vi "Queue Actor.vi"(8 "Queue Caller":map{string, refnum<data-value>}(c390), 9 "Queue of Queue Self":refnum<queue>, 10 "Queue Self Alias":string, 11 "Queue Actor":refnum<class "Queue Actor.lvclass">) -> ()   [LabVIEW 2021, in "jettl Queue Actor.lvlib" / "jettl Queue Actor.lvclass"]
uses:
  jettl Queue Actor.lvclass
  jettl Queue Actor.lvlib
  Actor/Msgs/Queue Last Ack/Queue Last Ack Msg/Queue Last Ack Msg.lvclass
  Actor/Msgs/Setup/Setup Msg/Setup Msg.lvclass
  Actor/Queue Actor/Queue Actor.lvclass
  Actor/Msg/Msg.lvclass
  C:/git/jettl/src/Actor/Actor/Actor.lvclass
  C:/git/jettl/src/Actor/Msgs/Setup/Setup/Setup.lvclass
  C:/git/jettl/src/Actor/Msgs/Teardown/Teardown/Teardown.lvclass
  C:/git/jettl/src/Actor/Queue Actor/Queue Actor.lvclass
  C:/git/jettl/src/Actor/Msgs/Event Create/Event Create/Event Create.lvclass
  C:/git/jettl/src/Actor/Msgs/Event Last Ack/Event Last Ack/Event Last Ack.lvclass
  C:/git/jettl/src/Actor/Msgs/Queue Create/Queue Create/Queue Create.lvclass
  C:/git/jettl/src/Actor/Msgs/Queue Last Ack/Queue Last Ack/Queue Last Ack.lvclass
  C:/git/jettl/src/jettl/jettl Queue Actor/jettl Queue Actor/jettl Queue Actor.lvclass
  C:/git/jettl/src/Actor/Msgs/Setup/Setup Msg/Setup Msg.lvclass
  C:/git/jettl/src/Actor/Msg/Msg.lvclass
  C:/git/jettl/src/Actor/Msgs/Queue Last Ack/Queue Last Ack Msg/Queue Last Ack Msg.lvclass
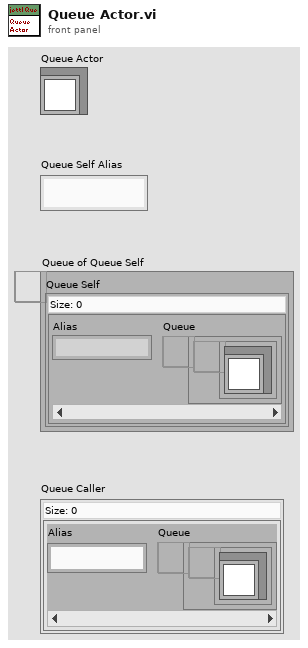
[diagram p1: front panel]
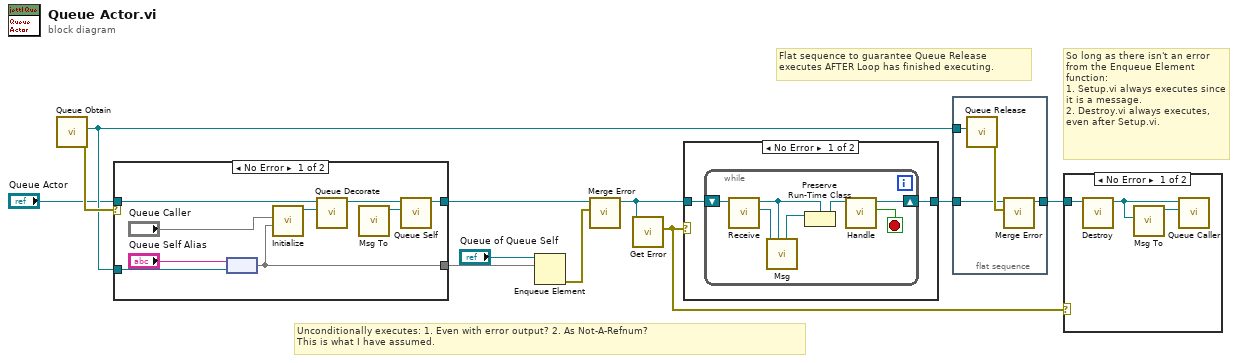
[diagram p0: block diagram]
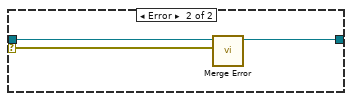
[diagram p3: hidden frame]
diagram:
  # "Flat sequence to guarantee Queue Release executes AFTER Loop has finished executing."
  # "Unconditionally executes: 1. Even with error output? 2. As Not-A-Refnum?\nThis is what I have assumed."
  # "So long as there isn't an error from the Enqueue Element function:\n1. Setup.vi always executes since it is a message.\n2. Destroy.vi always executes, even after Setup.vi."
  n1 = call "Queue Obtain.vi"() -> ("error out"=w11:errorcluster, "Queue"=w6:refnum<data-value>)  [unwired: 10 in]
  n2 = case shown="No Error" w11 {
    selector: w11 -> [_ w22]
    tunnel: [w19 w23] -> w4
    tunnel: "Queue Actor" -> [w18 w21]
    tunnel: w6 -> [w14 _]
    tunnel: [w12 _] -> w3
    frame No Error {
      n3 = node("Queue Self Alias", w14) -> (w12:map{string, refnum<data-value>})
      n4 = call "Initialize.vi"("Queue Self"=w12, "Queue Caller"="Queue Caller") -> ("jettl Queue Actor out"=w16:refnum<class "jettl Queue Actor.lvclass">)  [unwired: 9 in]
      n5 = call-dynamic "Queue Decorate.vi"("Queue Actor"=w16, "Queue Actor in"=w18) -> ("Queue Actor out"=w17:refnum<class "Queue Actor.lvclass">)  [unwired: 9 in]
      n6 = call "Msg To.vi"() -> ("Setup Msg out"=w20:refnum<class "Setup Msg.lvclass">)  [unwired: 11 in]
      n7 = call-dynamic "Queue Self.vi"("Msg"=w20, "Actor in"=w17) -> ("Actor out"=w19:refnum<class "Queue Actor.lvclass">)  [unwired: 9 in]
    }
    frame Error {
      n8 = call-dynamic "Merge Error.vi"("Error"=w22, "Set Error in"=w21) -> ("Set Error out"=w23:refnum<class "Queue Actor.lvclass">)  [unwired: 9 in]
    }
  }
  n9 = Enqueue Element(queue="Queue of Queue Self", element=w3) -> (error out=w8:errorcluster)  [unwired: 2 in, 2 out]
  n10 = call-dynamic "Merge Error.vi"("Error"=w8, "Set Error in"=w4) -> ("Set Error out"=w9:refnum<class "Queue Actor.lvclass">)  [unwired: 9 in]
  n11 = call-dynamic "Get Error.vi"("Actor in"=w9) -> ("Error"=w2:errorcluster)  [unwired: 10 in]
  n12 = case shown="No Error" w2 {
    tunnel: w9 -> [w25 w33]
    tunnel: [w24 w33] -> w1
    frame No Error {
      n13 = while {
        shift-right: [w32] -> w24
        shift-left: w25 -> [w28]
        stop <- w31 stop-if-true
        n14 = call-dynamic "Receive.vi"("Queue Actor in"=w28) -> ("Msg"=w26:refnum<class "Msg.lvclass">, "Queue Actor out"=w27:refnum<class "Queue Actor.lvclass">)  [unwired: 9 in]
        n15 = call-dynamic "Msg.vi"("Actor in"=w27, "Msg in"=w26) -> ("Actor out"=w30:refnum<class "Actor.lvclass">)  [unwired: 9 in]
        n16 = Preserve Run-Time Class(object in=w30, 2:w27) -> (object out=w29:refnum<class "Queue Actor.lvclass">)  [unwired: 1 in, 1 out]
        n17 = call-dynamic "Handle.vi"("Actor in"=w29) -> ("Destroy?"=w31:bool, "Actor out"=w32:refnum<class "Queue Actor.lvclass">)  [unwired: 9 in]
      }
    }
    frame Error {
    }
  }
  n18 = flat-sequence {
    tunnel: w6 -> [w37]
    tunnel: [w36] -> w10
    tunnel: w1 -> [w34]
    frame #0 {
      n19 = call "Queue Release.vi"("Queue"=w37) -> ("error out"=w35:errorcluster)  [unwired: 10 in]
      n20 = call-dynamic "Merge Error.vi"("Error"=w35, "Set Error in"=w34) -> ("Set Error out"=w36:refnum<class "Queue Actor.lvclass">)  [unwired: 9 in]
    }
  }
  n21 = case shown="No Error" w2 {
    tunnel: w10 -> [w38 _]
    frame No Error {
      n22 = call-dynamic "Destroy.vi"("Actor in"=w38) -> ("Actor out"=w39:refnum<class "Queue Actor.lvclass">)  [unwired: 10 in]
      n23 = call "Msg To.vi"("Queue Actor"=w39) -> ("Queue Last Ack Msg out"=w40:refnum<class "Queue Last Ack Msg.lvclass">)  [unwired: 10 in]
      n24 = call-dynamic "Queue Caller.vi"("Msg"=w40, "Actor in"=w39) -> ()  [unwired: 9 in, 1 out]
    }
    frame Error {
    }
  }
